vi "add to query.vi"(8 "error in (no error)":errorcluster, 11 "address":string) -> (0 "error out":errorcluster, 2 "function return":bool, 3 "address out":string)   [LabVIEW 2015, in "XGL_DPP.lvlib"]
doc: "EXTERN DECLSPEC bool CALL_CONV add_to_query(char* address);"
uses:
  XGL_DPP.lvlib
  XGL_DPP.dll
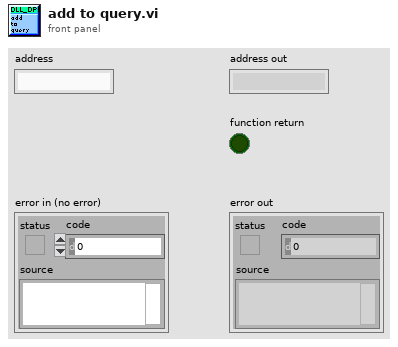
[diagram p1: front panel]
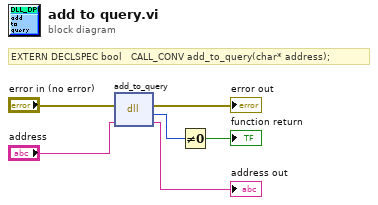
[diagram p0: block diagram]
diagram:
  # "EXTERN DECLSPEC bool   CALL_CONV add_to_query(char* address);"
  n1 = dll-call lib="D:/Users/XRF/Desktop/Dante_acquire4/libs/Dante/XGL_DPP.*" fn="add_to_query"(error in="error in (no error)", "address"="address") -> (error out=→"error out":errorcluster, "return type"=w5:u8, "address"=→"address out":string)  [unwired: 2 in, 1 out]
  n2 = Not Equal To 0?(x=w5) -> (x != 0?=→"function return":bool)
